vi "Dashboard Main.vi"() -> ()   [LabVIEW 2011]
uses:
  2012 Robot project FINAL/Dashboard Datatype.ctl
  <vilib>/Rock Robotics/WPI/DriverStation/WPI_DriverStationDigitalData.ctl
  <vilib>/vision/NI_Vision_Development_Module.lvlib
panel:
  out "Autonomous Robot Field Spot":string
  out "Driver Control":bool
  out "Shooter Control":bool
  out "Has The Kicker\nRestored?":bool
  out "Can I Shoot?":bool
  out "Are There 3 Balls In?":bool
  out "Distance From Target":dbl
  out "Current Speed":dbl
  out "Speed Wanted":dbl
  in  "Viewer":enum32{"Camera Image"}(tab)
  out "Camera Image":T1(plugin-control)
  out "Dashboard Datatype Warning":string="Warning: The Dashboard Datatype used by the robot project and this dashboard do not match.\nSee diagram for more details."
  out "Robot IP Address":string
  out "Image Error Message":string="Timeout in Camera Communications"
  # "Communications"
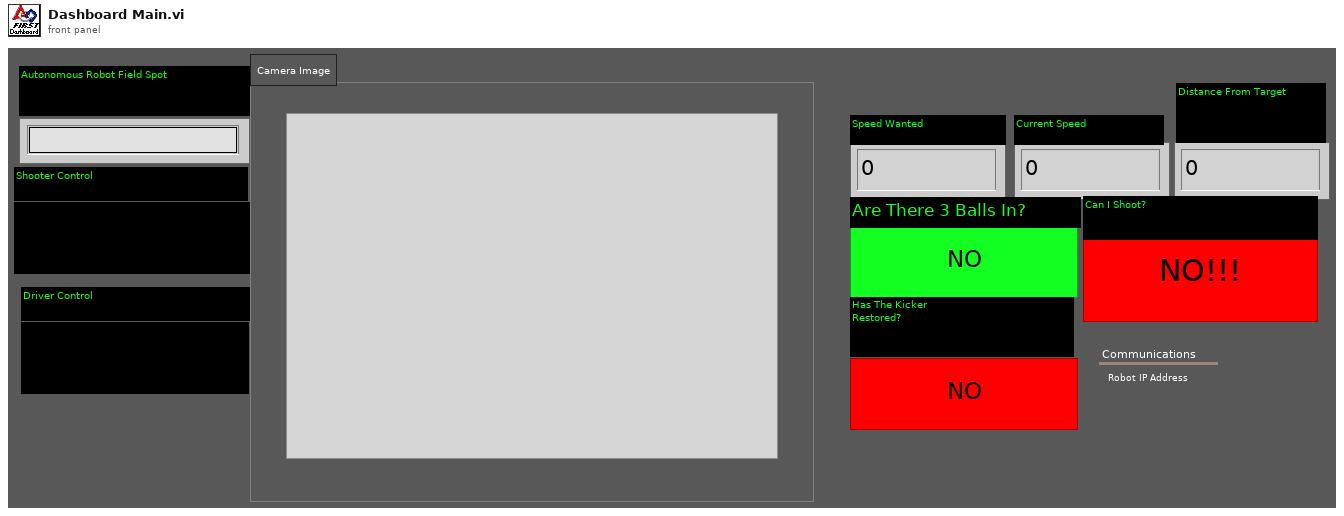
[diagram p1: front panel]
types:
  T1 = typedef "IMAQ Image.ctl" = refnum<image>
  T2 = typedef "Image Type" = u32
  T3 = typedef "Dashboard Datatype.ctl" = cluster{cluster{"AnalogModule[0]":cluster{"Channel[0]":sgl, "Channel[1]":sgl, "Channel[2]":sgl, "Channel[3]":sgl, "Channel[4]":sgl, "Channel[5]":sgl, "Channel[6]":sgl, "Channel[7]":sgl}, "AnalogModule[1]":cluster{"Channel[0]":sgl, "Channel[1]":sgl, "Channel[2]":sgl, "Channel[3]":sgl, "Channel[4]":sgl, "Channel[5]":sgl, "Channel[6]":sgl, "Channel[7]":sgl}}, cluster{"DigitalModule[0]":T4, "DigitalModule[1]":T4}, "SpeedWanted":dbl, "CurentSpeed":dbl, "UltrasonicDistance":dbl, "3Ball'sIn":bool, "Collector?":bool, "Kicker Restored?":bool, "InRange?":bool, "DriverControl":bool, "ShooterControl":bool, "WhereAmIString?":string}
  T4 = typedef "WPI_DriverStationDigitalData.ctl" = cluster{"Relay Fwd":u8, "Relay Rev":u8, "GPIO":u16, "GPIO_OE":u16, "PWM":cluster{"PWM[0]":u8, "PWM[1]":u8, "PWM[2]":u8, "PWM[3]":u8, "PWM[4]":u8, "PWM[5]":u8, "PWM[6]":u8, "PWM[7]":u8, "PWM[8]":u8, "PWM[9]":u8}}
  T5 = typedef "LVRectTypeDef.ctl" = cluster{"left":i16, "top":i16, "right":i16, "bottom":i16}
  T6 = cluster{"Competition mode":bool, "Robot Link":bool, "Autonomous":bool, "Enabled":bool, "E-Stop":bool}
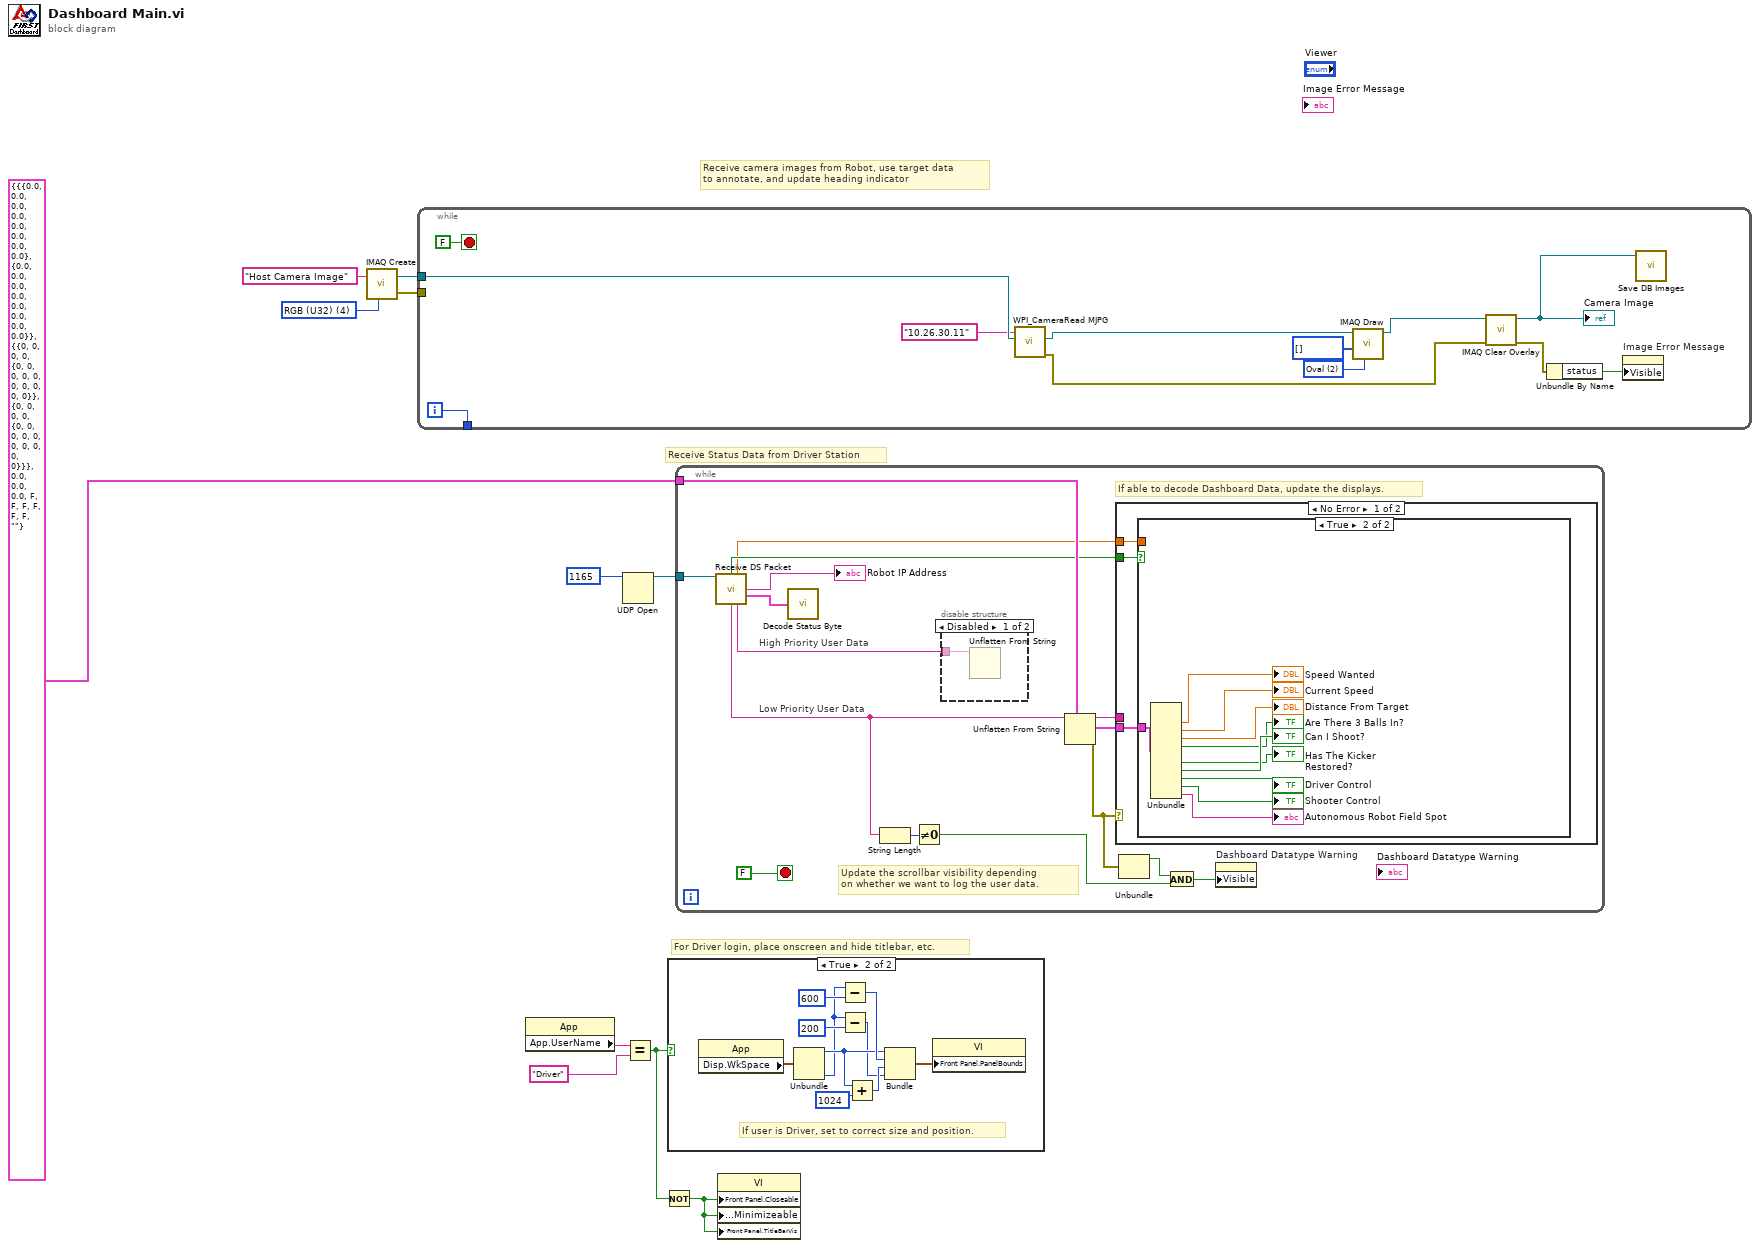
[diagram p0: block diagram]
diagram:
  w4 = T2 4 items=["Grayscale (U8)", "Grayscale (I16)", "Grayscale (SGL)", "Complex (CSG)", "RGB (U32)", "HSL (U32)", "RGB (U64)"] ("Image Type")
  # "For Driver login, place onscreen and hide titlebar, etc."
  # "Receive Status Data from Driver Station"
  # "Receive camera images from Robot, use target data\nto annotate, and update heading indicator"
  n1 = call "IMAQ Create"("Image Name"="Host Camera Image", "Image Type"=w4) -> ("New Image"=w2:T1, "error out"=w1:errorcluster)  [unwired: 2 in, 1 out]
  n2 = while {
    tunnel: w2 -> [w22]
    tunnel: w1 -> [_]
    tunnel: [w21] -> _
    i -> [w21]
    stop <- FALSE stop-if-true
    w13 = u16 2 items=["Line", "Rectangle", "Oval"] ("Shape to draw")
    n3 = call <vilib>:"WPI_CameraRead MJPG.vi"("Image"=w22, "address"="10.26.30.11") -> ("error out"=w12:errorcluster, "Image Out"=w20:T1)  [unwired: 8 in]
    n4 = call "IMAQ Draw"("Shape to draw"=w13, "Coordinates"=i32[] [], "Image Src"=w20) -> ("Image Dst Out"=w19:T1)  [unwired: 7 in, 1 out]
    n5 = call "IMAQ Clear Overlay"("error in (no error)"=w12, "Image"=w19) -> ("error out"=w18:errorcluster, "Image Out"=w16:T1)  [unwired: 1 in, 7 out]
    "Camera Image" <- w16
    n6 = Unbundle By Name(w18) -> ("status"=w17:bool)
    n7 = property on="Image Error Message" class="Str"("Visible"=w17) -> ()  [unwired: 2 in, 2 out]
    n8 = call "Save DB Images.vi"("Image"=w16) -> ()  [unwired: 2 in, 1 out]
  }
  n9 = property class="App"() -> ("App.UserName"=w8:string)  [unwired: 2 in, 2 out]
  n10 = UDP Open(11:u16 1165 ("port")) -> (port=w10:refnum<k16>)  [unwired: 2 in, 4 out]
  n11 = Equal?(x=w8, y="Driver") -> (x = y?=w7:bool)
  n12 = Not(x=w7) -> (.not. x?=w6:bool)
  n13 = case shown="True" w7 {
    frame False {
    }
    frame True {
      # "If user is Driver, set to correct size and position."
      n14 = property class="App"() -> ("Disp.WkSpace"=w33:T5)  [unwired: 2 in, 2 out]
      n15 = Unbundle(w33) -> ("left"=w28:i16, "bottom"=w24:i16)  [unwired: 2 out]
      n16 = Subtract(x=w24, y=600) -> (x-y=w30:i32)
      n17 = Subtract(x=w24, y=200) -> (x-y=w25:i32)
      n18 = Add(x=w28, y=1024) -> (x+y=w29:i32)
      n19 = Bundle("left"=w28, w30, w29, w25) -> (w32:cluster{"left":i16, i32, i32, i32})  [unwired: 1 out]
      n20 = property class="VI"("Front Panel.PanelBounds"=w32) -> ()  [unwired: 2 in, 2 out]
    }
  }
  n21 = while {
    tunnel: w10 -> [w47]
    tunnel: T3 {{"AnalogModule[0]"={"Channel[0]"=0.0, "Channel[1]"=0.0, "Channel[2]"=0.0, "Channel[3]"=0.0, "Channel[4]"=0.0, "Channel[5]"=0.0, "Channel[6]"=0.0, "Channel[7]"=0.0}, "AnalogModule[1]"={"Channel[0]"=0.0, "Channel[1]"=0.0, "Channel[2]"=0.0, "Channel[3]"=0.0, "Channel[4]"=0.0, "Channel[5]"=0.0, "Channel[6]"=0.0, "Channel[7]"=0.0}}, {"DigitalModule[0]"={"Relay Fwd"=0, "Relay Rev"=0, "GPIO"=0, "GPIO_OE"=0, "PWM"={"PWM[0]"=0, "PWM[1]"=0, "PWM[2]"=0, "PWM[3]"=0, "PWM[4]"=0, "PWM[5]"=0, "PWM[6]"=0, "PWM[7]"=0, "PWM[8]"=0, "PWM[9]"=0}}, "DigitalModule[1]"={"Relay Fwd"=0, "Relay Rev"=0, "GPIO"=0, "GPIO_OE"=0, "PWM"={"PWM[0]"=0, "PWM[1]"=0, "PWM[2]"=0, "PWM[3]"=0, "PWM[4]"=0, "PWM[5]"=0, "PWM[6]"=0, "PWM[7]"=0, "PWM[8]"=0, "PWM[9]"=0}}}, "SpeedWanted"=0.0, "CurentSpeed"=0.0, "UltrasonicDistance"=0.0, "3Ball'sIn"=FALSE, "Collector?"=FALSE, "Kicker Restored?"=FALSE, "InRange?"=FALSE, "DriverControl"=FALSE, "ShooterControl"=FALSE, "WhereAmIString?"=""} ("Dashboard Data") -> [w46]
    stop <- FALSE stop-if-true
    # "High Priority User Data"
    # "Low Priority User Data"
    # "Update the scrollbar visibility depending\non whether we want to log the user data."
    # "If able to decode Dashboard Data, update the displays."
    n22 = call "Receive DS Packet.vi"("Recv Socket"=w47) -> ("New Dashboard Data"=w44:bool, "Battery"=w35:sgl, "Robot IP Address"=→"Robot IP Address":string, "Status"=w48:T6, "Low Priority User Data"=w37:string, "High Priority User Data"=w36:string)  [unwired: 1 in, 8 out]
    n23 = call "Decode Status Byte.vi"("Status Byte"=w48) -> ()  [unwired: 2 out]
    n24 = String Length(string=w37) -> (length=w39:i32)
    n25 = Not Equal To 0?(x=w39) -> (x != 0?=w42:bool)
    n26 = disable-structure shown="Disabled" {
      disable-tunnel: w36 -> [w50 _]
      frame Disabled {
        n27 = Unflatten From String(binary string=w50) -> ()  [unwired: 2 in, 5 out]
      }
      frame Enabled {
      }
    }
    n28 = Unflatten From String(type=w46, binary string=w37) -> (rest of the binary string=w40:string, value=w34:T3, error out=w45:errorcluster)  [unwired: 1 in, 2 out]
    n29 = case shown="No Error" w45 {
      tunnel: w34 -> [w53 _]
      tunnel: w44 -> [w52 _]
      tunnel: w40 -> [_ _]
      tunnel: w35 -> [w51 _]
      frame No Error {
        n30 = case shown="True" w52 {
          tunnel: w53 -> [_ w63]
          tunnel: w51 -> [_ _]
          frame False {
            # "Don't update if the robot hasn't sent new data"
          }
          frame True {
            n31 = Unbundle(w63) -> ("SpeedWanted"=→"Speed Wanted":dbl, "CurentSpeed"=→"Current Speed":dbl, "UltrasonicDistance"=→"Distance From Target":dbl, "3Ball'sIn"=→"Are There 3 Balls In?":bool, "Kicker Restored?"=→"Has The Kicker\nRestored?":bool, "InRange?"=→"Can I Shoot?":bool, "DriverControl"=→"Driver Control":bool, "ShooterControl"=→"Shooter Control":bool, "WhereAmIString?"=→"Autonomous Robot Field Spot":string)  [unwired: 3 out]
          }
        }
      }
      frame Error {
        # "Your datatypes don't match. The Dashboard Datatype.ctl in your Robot project\nand the big constant to the left of the loop need to match."
      }
    }
    n32 = Unbundle(w45) -> ("status"=w41:bool)  [unwired: 2 out]
    n33 = And(x=w41, y=w42) -> (x .and. y?=w43:bool)
    n34 = property on="Dashboard Datatype Warning" class="Str"("Visible"=w43) -> ()  [unwired: 2 in, 2 out]
  }
  n35 = property class="VI"("Front Panel.Closeable"=w6, "Front Panel.Minimizeable"=w6, "Front Panel.TitleBarVis"=w6) -> ()  [unwired: 2 in, 2 out]
